vi "AB_Engine_Variable_Deployment_IncludedFiles.vi"(8 "error in (no error)":errorcluster, 10 "shared variable libraries only":bool, 11 "source items":refnum<class "AB_Source.lvclass">[](array[class])) -> (0 "error out":errorcluster, 1 "Included VIs":path[](array[path]), 3 "Included libraries":path[](array[path]))   [LabVIEW 2020]
uses:
  <vilib>/AppBuilder/AB_Classes/Source/AB_Source.lvclass
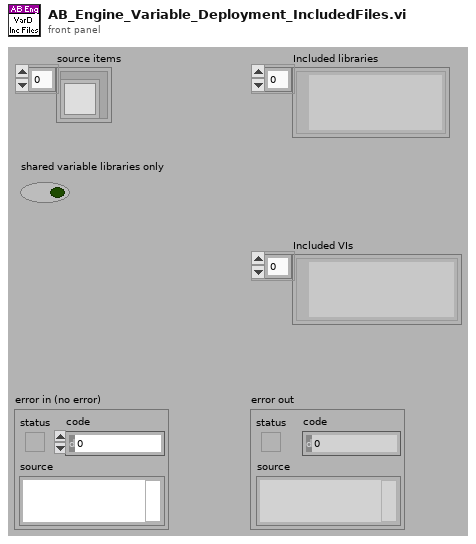
[diagram p1: front panel]
types:
  T1 = typedef "AB_Source.ctl" = cluster{"path":path, "itemID":string, "parentIndex":i32, "sourceInclusion":T2, "destinationIndex":i32, "properties":T3[], "newName":string, "lvfile":bool, "valid":bool, "eng_inBuild":bool, "eng_isNonVILink":bool, "Amalgamation":bool, "Amalgamation Piece":bool, "eng_delimitedName":string, "preventRename":bool}
  T2 = typedef "AB_Source_Inclusion.ctl" = enum16{"IncludeIfReferenced", "Include", "Exclude", "TopLevel"}
  T3 = typedef "AB_Source_Properties.ctl" = cluster{"sourcePropertyType":T4, "value":variant}
  T4 = typedef "AB_Source_Property_Type.ctl" = enum16{"Remove block diagram", "Remove front panel", "Password", "Window has title bar", "Show menu bar", "Show vertical scroll bar", "Show horizontal scroll bar", "Show toolbar", "Show Abort button", "Show fp when called", "Window behavior", "Allow user to close window", "Window run-time position", "Run when opened", "Allow debugging", "Auto error handling", "Generate guard code", "Use stack variables", "Expression folding", "Integer only", "Inline subVI"}
  T5 = enum16{"Single-Process", "Network-Published", "Time-Triggered", "Industrial"}
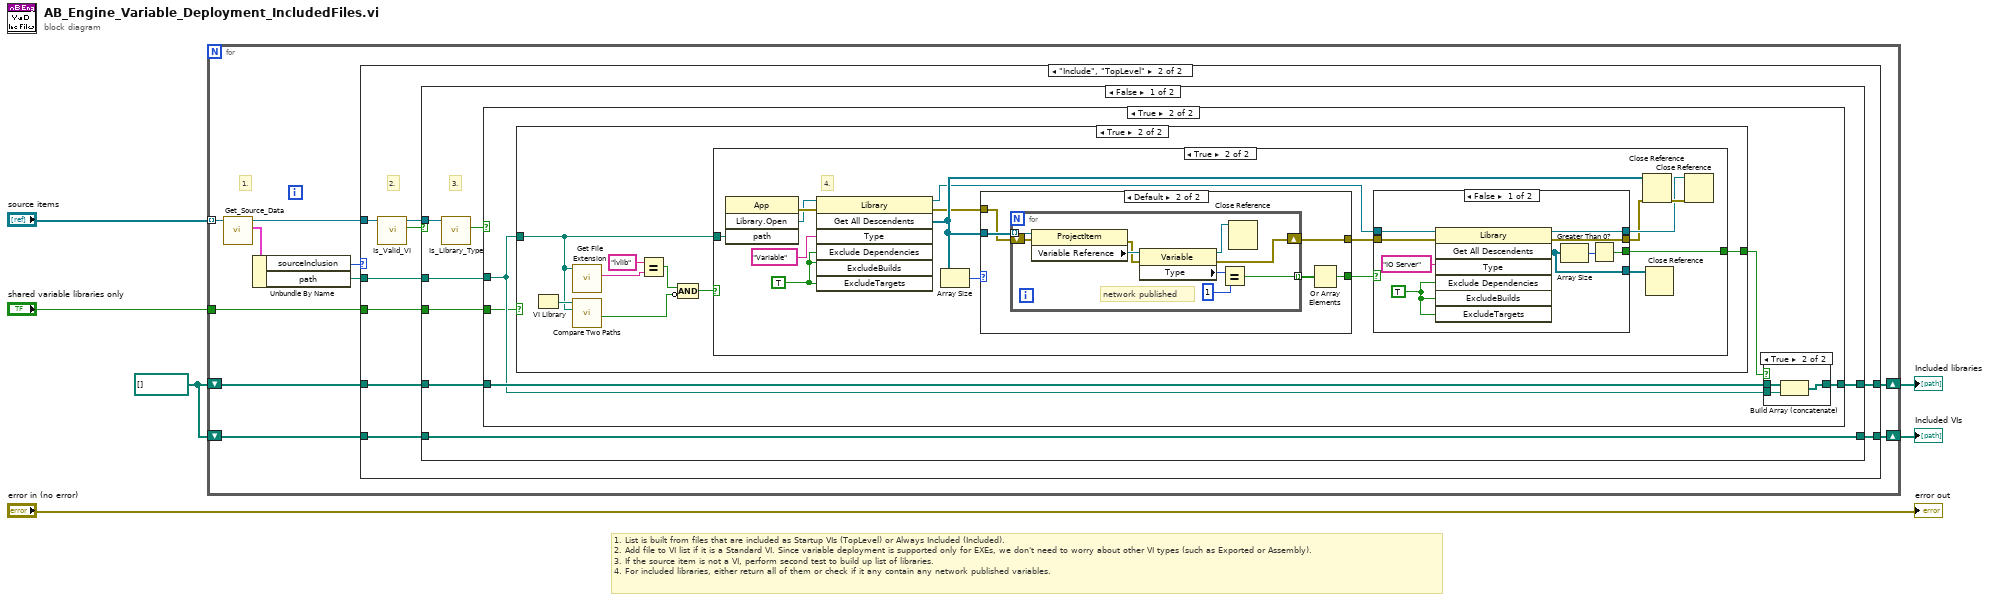
[diagram p0: block diagram]
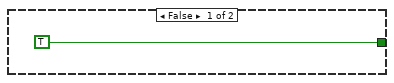
[diagram p4: hidden frame]
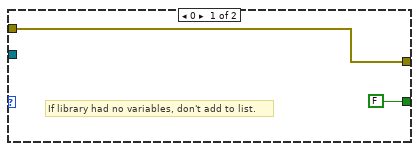
[diagram p7: hidden frame]
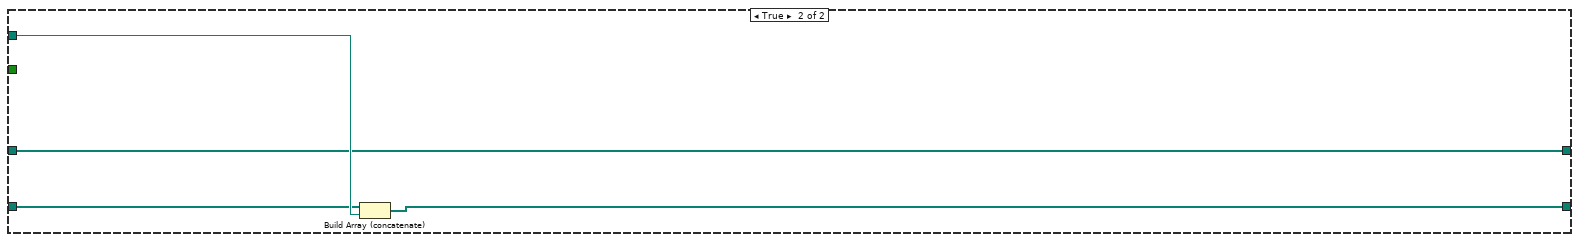
[diagram p9: hidden frame]
diagram:
  w4 = path[] []
  # "1. List is built from files that are included as Startup VIs (TopLevel) or Always Included (Included).\n2. Add file to VI list if it is a Standard VI. Since variable deployment is supported only for EXEs, we don't need to worry about other VI types (such as Exported or Assembly).\n3. If the source item is not a VI, perform second test to build up list of libraries.\n4. For included libraries, either return all of them or check if it any contain any network published variables."
  n1 = for {
    tunnel: "source items" -> [w12] mode=indexing
    shift-right: [w16] -> w6
    shift-left: w4 -> [w15]
    shift-right: [w13] -> w3
    shift-left: w4 -> [w14]
    tunnel: "shared variable libraries only" -> [w7]
    # "1."
    n2 = call <vilib>:"Get_Source_Data.vi"("Class in"=w12) -> ("data"=w10:T1, "Class out"=w11:refnum<class "AB_Source.lvclass">)  [unwired: 1 in, 8 out]
    n3 = Unbundle By Name(w10) -> ("sourceInclusion"=w9:T2, "path"=w8:path)
    n4 = case shown="\"Include\", \"TopLevel\"" w9 {
      tunnel: [w17 w27] -> w16
      tunnel: w15 -> [w17 w26]
      tunnel: w14 -> [w18 w25]
      tunnel: [w18 w24] -> w13
      tunnel: w11 -> [_ w23]
      tunnel: w8 -> [_ w20]
      tunnel: w7 -> [_ w19]
      frame Default {
      }
      frame "Include", "TopLevel" {
        # "2."
        n5 = call-dynamic "Is_Valid_VI.vi"("AB_Source in"=w23) -> ("VI"=w21:bool, "AB_Source out"=w22:refnum<class "AB_Source.lvclass">)  [unwired: 2 in, 7 out]
        n6 = case shown="False" w21 {
          tunnel: w20 -> [w33 w101]
          tunnel: [w34 w100] -> w27
          tunnel: w26 -> [w34 w99]
          tunnel: w22 -> [w30 _]
          tunnel: w25 -> [w32 w98]
          tunnel: [w31 w98] -> w24
          tunnel: w19 -> [w28 _]
          frame False {
            # "3."
            n7 = call-dynamic "Is_Library_Type.vi"("AB_Source in"=w30) -> ("library type"=w29:bool)  [unwired: 1 in, 9 out]
            n8 = case shown="True" w29 {
              tunnel: w33 -> [_ w39]
              tunnel: w32 -> [w35 w40]
              tunnel: [w35 w38] -> w31
              tunnel: w28 -> [_ w36]
              frame False {
              }
              frame True {
                n9 = case shown="True" w36 {
                  tunnel: w39 -> [_ w44]
                  tunnel: [TRUE w49] -> w37
                  frame False {
                  }
                  frame True {
                    n10 = VI Library() -> (path=w48:path)
                    n11 = call <vilib>:"Get File Extension.vi"("file"=w44) -> ("lowercase file extension"=w42:string)  [unwired: 6 in, 4 out]
                    n12 = call <vilib>:"Compare Two Paths.vi"("Path 2"=w44, "Path 1"=w48) -> ("Path 2 Relative to Path 1?"=w45:bool)  [unwired: 6 in, 3 out]
                    n13 = Equal?(x="lvlib", y=w42) -> (x = y?=w46:bool)
                    n14 = Compound Arithmetic op=AND(w46, invert w45) -> (w43:bool)
                    n15 = case shown="True" w43 {
                      tunnel: [_ w52] -> w49
                      tunnel: w44 -> [_ w50]
                      frame False {
                      }
                      frame True {
                        w63 = TRUE
                        # "4."
                        n16 = invoke class="App" method="Library.Open"("path"=w50) -> (error out=w65:errorcluster, "Open Library"=w64:refnum<vi>)  [unwired: 3 in, 2 out]
                        n17 = invoke class="Library" method="Get All Descendents"(reference=w64, error in=w65, "Type"="Variable", "Exclude Dependencies"=w63, "ExcludeBuilds"=w63, "ExcludeTargets"=w63) -> (reference out=w55:refnum<vi>, error out=w58:errorcluster, "All Descendents"=w59:refnum<vi>[])  [unwired: 1 in, 4 out]
                        n18 = Array Size(array=w59) -> (size(s)=w60:i32)
                        n19 = case shown="Default" w60 {
                          tunnel: w59 -> [_ w84]
                          tunnel: [FALSE w80] -> w57
                          tunnel: w58 -> [w79 w83]
                          tunnel: [w79 w82] -> w56
                          frame 0 {
                            # "If library had no variables, don't add to list."
                          }
                          frame Default {
                            n20 = for {
                              tunnel: w84 -> [w93] mode=indexing
                              shift-right: [w88] -> w82
                              shift-left: w83 -> [w92]
                              tunnel: [w85] -> w81 mode=indexing
                              # "network published"
                              n21 = property class="ProjectItem"(reference=w93, error in=w92) -> (error out=w90:errorcluster, "Variable Reference"=w91:refnum<vi>)  [unwired: 1 out]
                              n22 = property class="Variable"(reference=w91, error in=w90) -> (reference out=w89:refnum<vi>, error out=w88:errorcluster, "Type"=w87:T5)
                              n23 = Equal?(x=w87, y=u16 1) -> (x = y?=w85:bool)
                              n24 = Close Reference(reference=w89) -> ()  [unwired: 1 in, 1 out]
                            }
                            n25 = Or Array Elements(Boolean array=w81) -> (logical OR=w80:bool)
                          }
                        }
                        n26 = case shown="False" w57 {
                          selector: w57 -> [_ w77]
                          tunnel: [w69 w77] -> w52
                          tunnel: w55 -> [w74 w76]
                          tunnel: w56 -> [w73 w75]
                          tunnel: [w68 w76] -> w54
                          tunnel: [w67 w75] -> w53
                          tunnel: [w66 _] -> w51
                          frame False {
                            w71 = TRUE
                            n27 = invoke class="Library" method="Get All Descendents"(reference=w74, error in=w73, "Type"="IO Server", "Exclude Dependencies"=w71, "ExcludeBuilds"=w71, "ExcludeTargets"=w71) -> (reference out=w68:refnum<vi>, error out=w67:errorcluster, "All Descendents"=w66:refnum<vi>[])  [unwired: 1 in, 4 out]
                            n28 = Array Size(array=w66) -> (size(s)=w70:i32)
                            n29 = Greater Than 0?(x=w70) -> (x > 0?=w69:bool)
                          }
                          frame True {
                          }
                        }
                        n30 = Close Reference(reference=w59, error in (no error)=w53) -> (error out=w61:errorcluster)
                        n31 = Close Reference(reference=w51) -> ()  [unwired: 1 in, 1 out]
                        n32 = Close Reference(reference=w54, error in (no error)=w61) -> ()  [unwired: 1 out]
                      }
                    }
                  }
                }
                n33 = case shown="True" w37 {
                  tunnel: w40 -> [w94 w97]
                  tunnel: w39 -> [_ w96]
                  tunnel: [w94 w95] -> w38
                  frame False {
                  }
                  frame True {
                    n34 = Build Array (concatenate)(w97, w96) -> (w95:path[])
                  }
                }
              }
            }
          }
          frame True {
            n35 = Build Array (concatenate)(w99, w101) -> (w100:path[])
          }
        }
      }
    }
  }
  "Included VIs" <- w6
  "Included libraries" <- w3
  "error out" <- "error in (no error)"
